vi "Write Error.vi"(8 "Error In":errorcluster, 11 "Error to be logged":T1) -> (0 "Error Out":errorcluster)   [LabVIEW 2023, in "Error Manager.lvlib" / "Error Log.lvclass"]
doc: "This VI logs the contents of a LabVIEW error to the Error Log file."
uses:
  Error Log.lvclass
  Error to be logged (cluster).ctl
  Error Type (enum).ctl
panel:
  out "Number of characters":i32
  out "Text written to log":string
  # "Input\nInputs to the VI"
  # "Development\nControls or indicators that are useful for development or testing, but which are not outputs of the VI."
  # "Output\nOutputs of the VI"
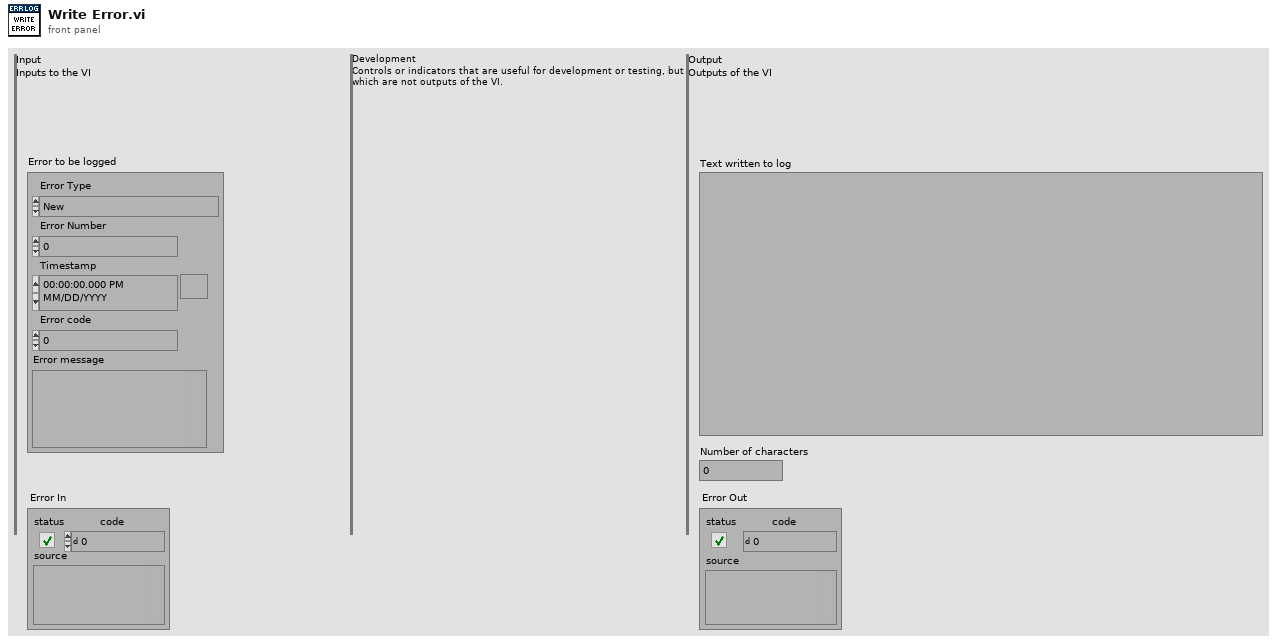
[diagram p1: front panel]
types:
  T1 = typedef "Error Manager.lvlib/Error Log.lvclass/Error to be logged (cluster).ctl" = cluster{"Error Type":T2, "Error Number":i32, "Timestamp":timestamp, "Error code":i32, "Error message":string}
  T2 = typedef "Error Manager.lvlib/Error Log.lvclass/Error Type (enum).ctl" = enum16{"New", "Identical to last logged error"}
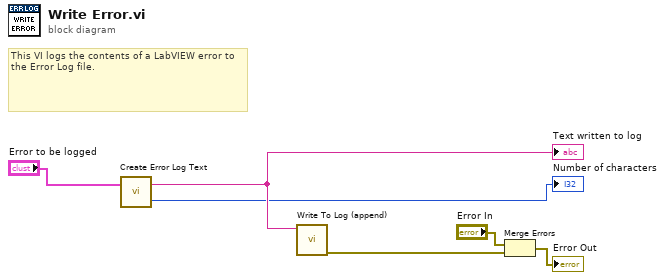
[diagram p0: block diagram]
diagram:
  # "This VI logs the contents of a LabVIEW error to the Error Log file."
  n1 = call "Create Error Log Text.vi"("Error to be logged"="Error to be logged") -> ("Number of characters"=→"Number of characters":i32, "Text to be written to error log file"=w2:string)  [unwired: 1 in]
  "Text written to log" <- w2
  n2 = call "Write To Log (append).vi"("Text to write"=w2) -> ("error out"=w4:errorcluster)  [unwired: 10 in]
  n3 = Merge Errors("Error In", w4) -> (→"Error Out":errorcluster)
